vi "Generate Doc URL.vi"(9 "Method Name":string, 10 "Owning Entity Name":string, 11 "URL Format":string) -> (2 "Final URL":string)   [LabVIEW 2014]
doc: "Copyright (c) 2018 Sze Howe Koh\n\nThis Source Code Form is subject to the terms of the Mozilla Public License, v. 2.0. If a copy of the MPL was not distributed with this file, You can obtain one at http://mozilla.org/MPL/2.0/."
uses:
  <vilib>/regexp/Match Regular Expression.xnode
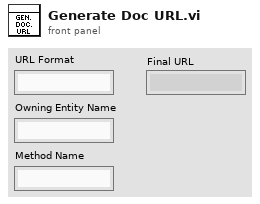
[diagram p1: front panel]
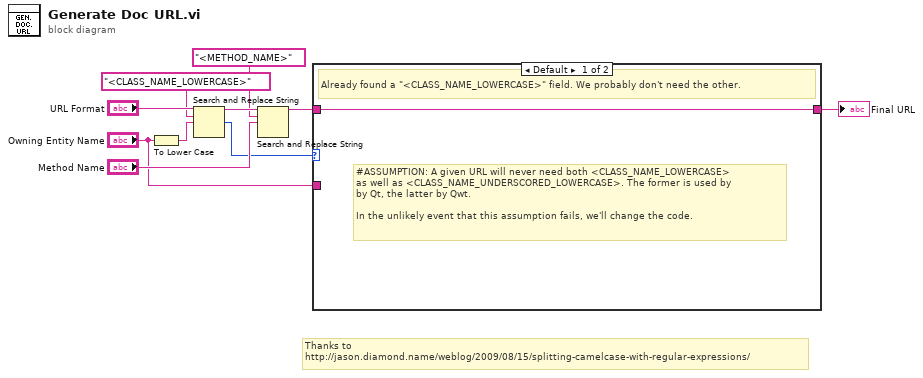
[diagram p0: block diagram]
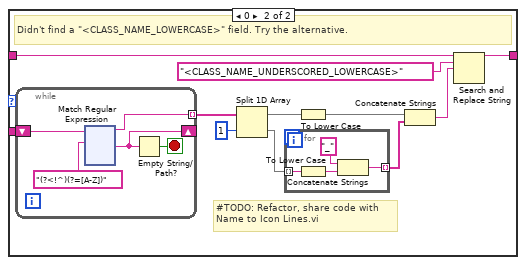
[diagram p2: hidden frame]
diagram:
  # "Thanks to\nhttp://jason.diamond.name/weblog/2009/08/15/splitting-camelcase-with-regular-expressions/"
  n1 = To Lower Case(string="Owning Entity Name") -> (all lower case string=w1:string)
  n2 = Search and Replace String(input string="URL Format", search string="<CLASS_NAME_LOWERCASE>", replace string=w1) -> (result string=w9:string, number of replacements=w3:i32)  [unwired: 5 in, 2 out]
  n3 = Search and Replace String(input string=w9, search string="<METHOD_NAME>", replace string="Method Name") -> (result string=w5:string)  [unwired: 5 in, 3 out]
  n4 = case shown="Default" w3 {
    tunnel: "Owning Entity Name" -> [_ w22]
    tunnel: w5 -> [w11 w17]
    tunnel: [w11 w14] -> w4
    frame Default {
      # "#ASSUMPTION: A given URL will never need both <CLASS_NAME_LOWERCASE>\nas well as <CLASS_NAME_UNDERSCORED_LOWERCASE>. The former is used by\nby Qt, the latter by Qwt.\n\nIn the unlikely event that this assumption fails, we'll change the code."
      # "Already found a \"<CLASS_NAME_LOWERCASE>\" field. We probably don't need the other."
    }
    frame 0 {
      # "#TODO: Refactor, share code with\nName to Icon Lines.vi"
      # "Didn't find a \"<CLASS_NAME_LOWERCASE>\" field. Try the alternative."
      n5 = while {
        shift-right: [w28] -> _
        shift-left: w22 -> [w29]
        tunnel: [w27] -> w19 mode=indexing
        stop <- w31 stop-if-true
        n6 = xnode "Match Regular Expression"("input string"=w29, "regular expression"="(?<!^)(?=[A-Z])") -> ("before match"=w27:string, "after match"=w28:string)  [unwired: 4 in, 3 out]
        n7 = Empty String/Path?(string/path=w28) -> (empty?=w31:bool)
      }
      n8 = Split 1D Array(array=w19, index=1) -> (first subarray=w13:string[], second subarray=w20:string[])
      n9 = for {
        tunnel: w20 -> [w26] mode=indexing
        tunnel: [w24] -> w18 mode=indexing
        n10 = To Lower Case(string=w26) -> (all lower case string=w25:string)
        n11 = Concatenate Strings("_" ("string"), w25) -> (w24:string)
      }
      n12 = To Lower Case(string=w13) -> (all lower case string=w12:string[])
      n13 = Concatenate Strings(w12, w18) -> (w15:string)
      n14 = Search and Replace String(input string=w17, search string="<CLASS_NAME_UNDERSCORED_LOWERCASE>", replace string=w15) -> (result string=w14:string)  [unwired: 5 in, 3 out]
    }
  }
  "Final URL" <- w4
